vi "BRig_dataMTrig_Solenoid_T_R.vi"() -> (2 "output_Solenoid_T_R":i32)   [LabVIEW 2014]
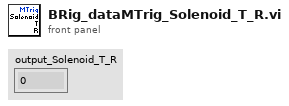
[diagram p1: front panel]
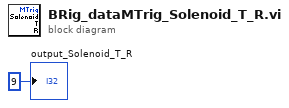
[diagram p0: block diagram]
diagram:
  "output_Solenoid_T_R" <- 9 ("output_iBlock")
